vi "VI Tree - numeric__ogtk.vi"   [LabVIEW 2009]
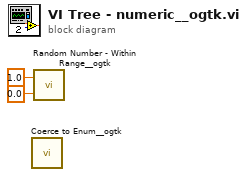
[diagram p0: block diagram]
diagram:
  n1 = call "Coerce to Enum__ogtk.vi"() -> ()  [unwired: 1 in]
  n2 = call "Random Number - Within Range__ogtk.vi"("High (1.00)"=1.0, "Low (0.00)"=0.0) -> ()  [unwired: 3 in, 1 out]
